vi "HomeUIRef.vi"(8 "error in (no error)":errorcluster, 11 "Controller in":refnum<class "Controller.lvclass">) -> (0 "error out":errorcluster, 2 "VIRef":refnum<vi>, 3 "Controller out":refnum<class "Controller.lvclass">)   [LabVIEW 2020, in "UIContainer.lvlib" / "Controller.lvclass"]
uses:
  Controller.lvclass
  Controller.lvclass/Controller.ctl
  UIHome/Controller/Controller.lvclass
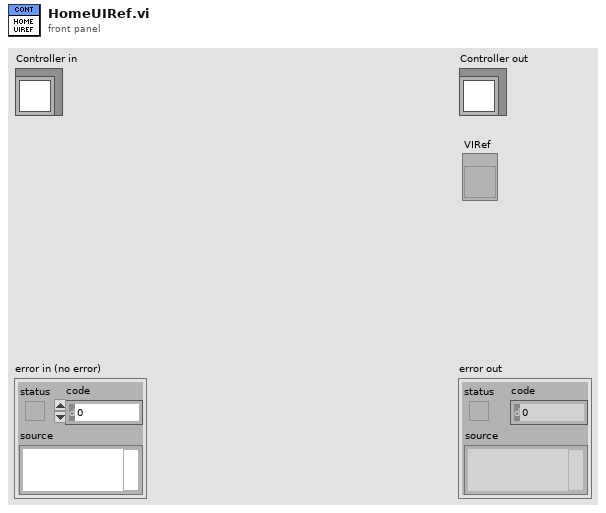
[diagram p1: front panel]
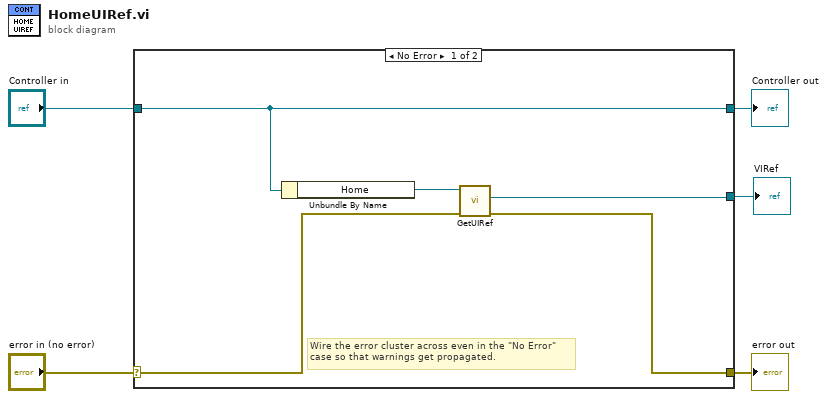
[diagram p0: block diagram]
diagram:
  n1 = case shown="No Error" "error in (no error)" {
    selector: "error in (no error)" -> [w8 w12]
    tunnel: [w7 w12] -> w4
    tunnel: [w10 w11] -> w2
    tunnel: "Controller in" -> [w10 w11]
    tunnel: [w6 _] -> w1
    frame No Error {
      # "Wire the error cluster across even in the \"No Error\"\ncase so that warnings get propagated."
      n2 = Unbundle By Name(w10) -> ("Home"=w9:refnum<class "Controller.lvclass">)
      n3 = call "GetUIRef.vi"("error in (no error)"=w8, "Controller in"=w9) -> ("error out"=w7:errorcluster, "VIRef"=w6:refnum<vi>)  [unwired: 7 in, 1 out]
    }
    frame Error {
    }
  }
  "error out" <- w4
  "Controller out" <- w2
  "VIRef" <- w1
